vi "ReadGlobalVars.vi"() -> (0 "Current Position":dbl[](array[numeric]))   [LabVIEW 2013]
uses:
  GlobalVars.vi
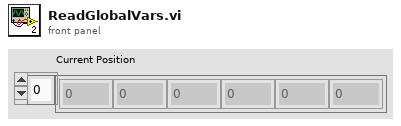
[diagram p1: front panel]
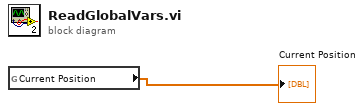
[diagram p0: block diagram]
diagram:
  n1 = global read "GlobalVars.vi" "Current Position"() -> (→"Current Position":dbl[])
